vi "Reset.vi"(8 "error in (no error)":errorcluster, 11 "AODAcq in":refnum<class "AODAcq.lvclass">) -> (0 "error out":errorcluster, 3 "AODAcq out":refnum<class "AODAcq.lvclass">)   [LabVIEW 2012, in "AODAcq.lvclass"]
uses:
  AODAcq.lvclass
  <vilib>/Utility/error.llb/Error Cluster From Error Code.vi
  <vilib>/rvi/errors/niLvFpgaAdjustHostInterfaceError.vi
  Program Files (x86)/National Instruments/LabVIEW 2012/Targets/NI/FPGA/StockFPGA_IntfPrivate/ScriptTemplates/StockFPGA_PlugInRead32.vi
  <vilib>/rvi/interface/nirviReadWriteControl/nirviReadWriteControl.xnode
  FPGA_Control/AODRef.ctl
  FPGA Bitfiles/AodScanner_FPGATarget_AODControl(FPGA)_HzWc4w5qqfg.lvbitx
  <vilib>/rvi/interface/nirviMethod/nirviMethod.xnode
  NiFpgaLv.dll
  <vilib>/FPGAPlugInAG/PXIe-7965R/niLvFpga_Read32_PXIe-7965R.vi
  <vilib>/rvi/interface/nirviReadWriteControl/niFpgaRWControlAccessTimeoutTemplate.vi
  <vilib>/FPGAPlugInAG/PXIe-7965R/niLvFpga_ReadFifo_PXIe-7965R.vi
  <vilib>/rvi/errors/niLvFpgaMergeErrorWithErrorCode.vi
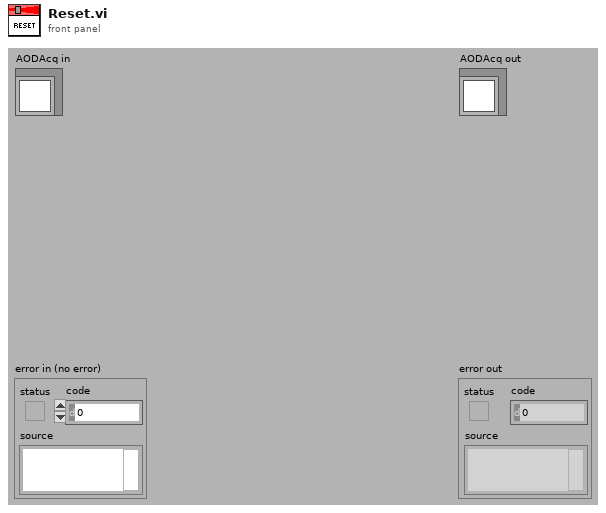
[diagram p1: front panel]
types:
  T1 = typedef "AODRef.ctl" = refnum<k20>
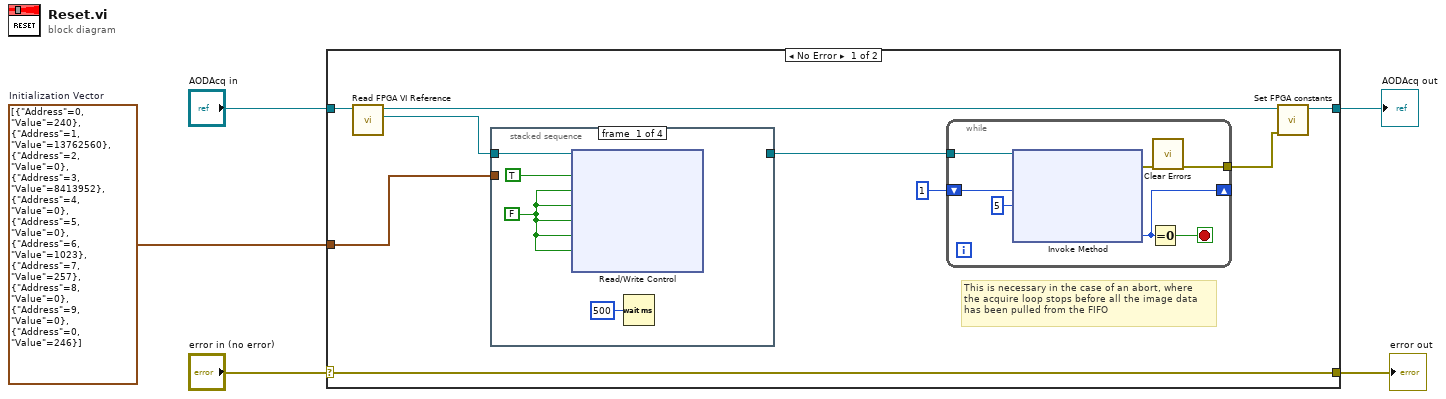
[diagram p0: block diagram]
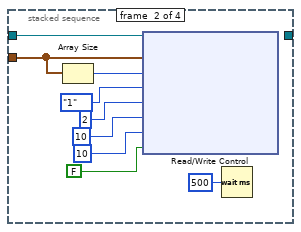
[diagram p2: hidden frame]
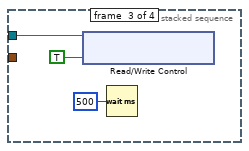
[diagram p3: hidden frame]
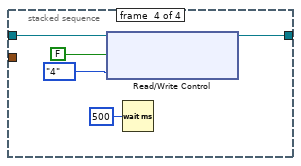
[diagram p4: hidden frame]
diagram:
  w1 = cluster{"Address":u8, "Value":u32}[] [{"Address"=0, "Value"=240}, {"Address"=1, "Value"=13762560}, {"Address"=2, "Value"=0}, {"Address"=3, "Value"=8413952}, {"Address"=4, "Value"=0}, {"Address"=5, "Value"=0}, {"Address"=6, "Value"=1023}, {"Address"=7, "Value"=257}, {"Address"=8, "Value"=0}, {"Address"=9, "Value"=0}, {"Address"=0, "Value"=246}]  # Initialization Vector
  n1 = case shown="No Error" "error in (no error)" {
    selector: "error in (no error)" -> [w14 w44]
    tunnel: [w14 w44] -> w4
    tunnel: [w7 w43] -> w2
    tunnel: "AODAcq in" -> [w10 w43]
    tunnel: w1 -> [w12 _]
    frame No Error {
      # "This is necessary in the case of an abort, where \nthe acquire loop stops before all the image data\nhas been pulled from the FIFO"
      n2 = call-dynamic "Read FPGA VI Reference.vi"("AODAcq in"=w10) -> ("FPGA VI Reference"=w11:T1, "AODAcq out"=w8:refnum<class "AODAcq.lvclass">)  [unwired: 8 in, 1 out]
      n3 = stacked-sequence {
        tunnel: w11 -> [w24 w32 w35 w40]
        tunnel: w12 -> [_ w31 _ _]
        tunnel: [_ _ _ w39] -> w9
        frame #0 {
          w23 = FALSE ("Abort")
          n4 = xnode "Read/Write Control"("FPGA VI Reference In"=w24, "Control.Reset"=TRUE ("Reset"), "Control.Stop"=w23, "Control.Points"=w23, "Control.Abort"=w23, "Control.Volume"=w23, "Comm.Write Register"=w23) -> ()  [unwired: 1 in, 3 out]
          n5 = Wait (ms)(milliseconds to wait=u32 500) -> ()  [unwired: 1 out]
        }
        frame #1 {
          n6 = Array Size(array=w31) -> (size(s)=w28:i32)
          n7 = xnode "Read/Write Control"("FPGA VI Reference In"=w32, "Comm.Write"=w31, "Comm.WriteSize"=w28, "Comm.CommLines"=enum16{"1", "2", "4"}."1" ("WriteSize"), "Comm.SclkDivider"=u32 2 ("ClockPause"), "Comm.UpdateIO time"=u32 10, "Comm.Pause"=u32 10, "Control.Reset"=FALSE ("Reset")) -> ()  [unwired: 1 in, 2 out]
          n8 = Wait (ms)(milliseconds to wait=u32 500) -> ()  [unwired: 1 out]
        }
        frame #2 {
          n9 = xnode "Read/Write Control"("FPGA VI Reference In"=w35, "Comm.Write Register"=TRUE ("Write Register")) -> ()  [unwired: 1 in, 2 out]
          n10 = Wait (ms)(milliseconds to wait=u32 500) -> ()  [unwired: 1 out]
        }
        frame #3 {
          n11 = xnode "Read/Write Control"("FPGA VI Reference In"=w40, "Comm.Write Register"=FALSE ("Write Register"), "Comm.CommLines"=enum16{"1", "2", "4"}."4" ("WriteSize")) -> ("FPGA VI Reference Out"=w39:T1)  [unwired: 1 in, 1 out]
          n12 = Wait (ms)(milliseconds to wait=u32 500) -> ()  [unwired: 1 out]
        }
      }
      n13 = while {
        tunnel: w9 -> [w21]
        shift-right: [w16] -> _
        shift-left: u32 1 ("Number of Elements") -> [w17]
        tunnel: [w15] -> w6
        stop <- w20 stop-if-true
        n14 = xnode "Invoke Method"("FPGA VI Reference In"=w21, "Number of Elements"=w17, "Timeout (ms)"=5) -> ("error out"=w18:errorcluster, "Elements Remaining"=w16:u32)  [unwired: 1 in, 2 out]
        n15 = Equal To 0?(x=w16) -> (x = 0?=w20:bool)
        n16 = call <vilib>:"Clear Errors.vi"("error in (no error)"=w18) -> ("error out"=w15:errorcluster)  [unwired: 6 in]
      }
      n17 = call-dynamic "Set FPGA constants.vi"("error in (no error)"=w6, "AODAcq in"=w8) -> ("AODAcq out"=w7:refnum<class "AODAcq.lvclass">)  [unwired: 8 in, 1 out]
    }
    frame Error {
    }
  }
  "error out" <- w4
  "AODAcq out" <- w2
